vi "Append Image Array.vi"(0 "index":i32, 1 "New Image Value":i32, 2 "Current Image Array":i32[](array[numeric])) -> (3 "Output Image Array":i32[](array[numeric]))   [LabVIEW 2018]
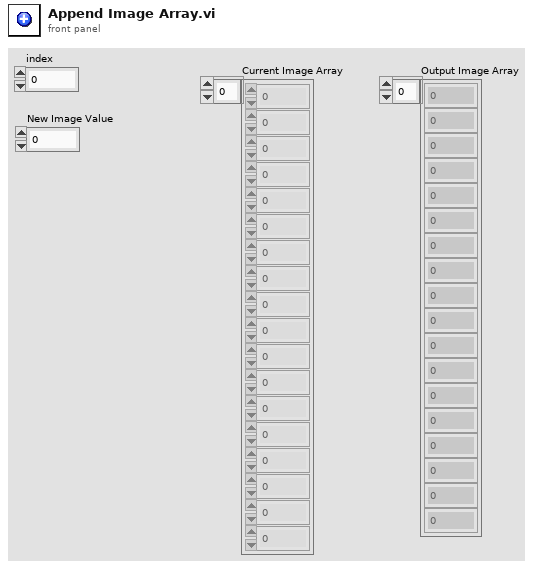
[diagram p1: front panel]
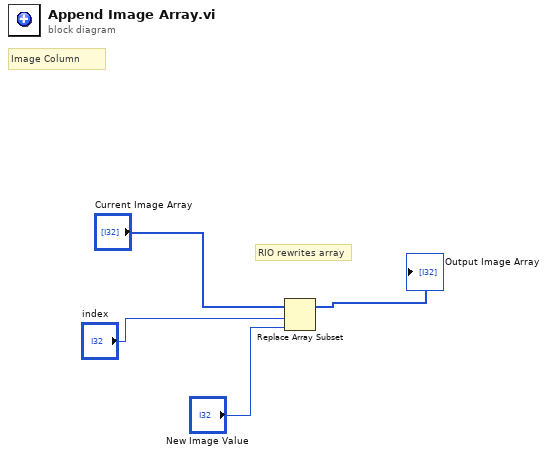
[diagram p0: block diagram]
diagram:
  # "Image Column"
  # "RIO rewrites array"
  n1 = Replace Array Subset(array="Current Image Array", new element="New Image Value", index="index") -> (→"Output Image Array":i32[])
